vi "Kickity.vi"(1 "btn 1":bool, 2 "i":i32) -> (0 "kick":bool)   [LabVIEW 2012]
panel:
  in  "offset":i32
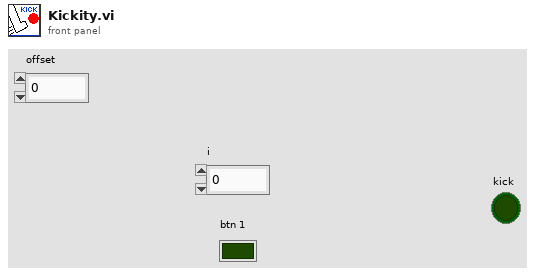
[diagram p1: front panel]
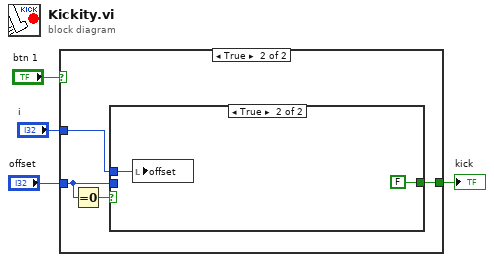
[diagram p0: block diagram]
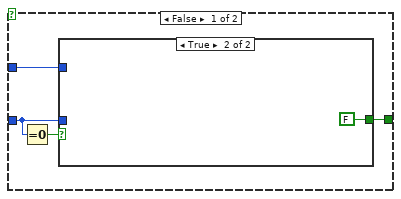
[diagram p2: hidden frame]
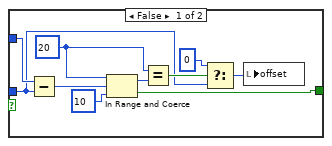
[diagram p3: hidden frame]
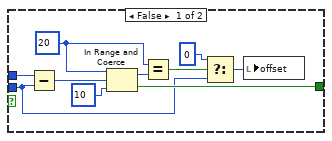
[diagram p4: hidden frame]
diagram:
  n1 = case shown="True" "btn 1" {
    tunnel: "i" -> [w6 w22]
    tunnel: "offset" -> [w7 w21]
    tunnel: [w5 w20] -> w1
    frame False {
      n2 = Equal To 0?(x=w7) -> (x = 0?=w8:bool)
      n3 = case shown="True" w8 {
        tunnel: w7 -> [w11 _]
        tunnel: w6 -> [w18 _]
        tunnel: [w13 FALSE] -> w5
        frame False {
          w15 = 20 ("upper limit")
          n4 = Subtract(x=w18, y=w11) -> (x-y=w17:i32)
          n5 = In Range and Coerce(upper limit=w15, x=w17, lower limit=10) -> (coerced(x)=w16:i32, In Range?=w13:bool)
          n6 = Equal?(x=w15, y=w16) -> (x = y?=w12:bool)
          n7 = Select(t=0, s=w12, f=w11) -> (s? t:f=w9:i32)
          n8 = local write "offset"(w9) -> ()
        }
        frame True {
        }
      }
    }
    frame True {
      n9 = Equal To 0?(x=w21) -> (x = 0?=w23:bool)
      n10 = case shown="True" w23 {
        tunnel: w22 -> [w33 w35]
        tunnel: w21 -> [w26 _]
        tunnel: [w28 FALSE] -> w20
        frame False {
          w31 = 20 ("upper limit")
          n11 = Subtract(x=w33, y=w26) -> (x-y=w29:i32)
          n12 = In Range and Coerce(upper limit=w31, x=w29, lower limit=10) -> (coerced(x)=w32:i32, In Range?=w28:bool)
          n13 = Equal?(x=w31, y=w32) -> (x = y?=w27:bool)
          n14 = Select(t=0, s=w27, f=w26) -> (s? t:f=w24:i32)
          n15 = local write "offset"(w24) -> ()
        }
        frame True {
          n16 = local write "offset"(w35) -> ()
        }
      }
    }
  }
  "kick" <- w1
